vi "运维调试_其他.vi"() -> ()   [LabVIEW 2016, in "其他.lvlib"]
uses:
  <vilib>/Utility/miscctls.llb/LVPointTypeDef.ctl
  <userlib>/_SmartBalloon/Balloon Generic/Aesthetics.ctl
  <userlib>/_SmartBalloon/Balloon/Text Balloon.lvclass
  C:/Program Files (x86)/National Instruments/LabVIEW 2016/user.lib/_SmartBalloon/Balloon Generic/Balloon.lvclass
  <userlib>/_SmartBalloon/Balloon/Init Balloon.vi
  <vilib>/ptbypt/NI_PtbyPt.lvlib
  WxMessage/wxpusher.lvlib
  <userlib>/_SmartBalloon/API/SmartBalloon Library.lvclass
  <userlib>/_SmartBalloon/Balloon Generic/Balloon.lvclass
  <vilib>/Utility/config.llb/NI_LVConfig.lvlib
  update/update/update.lvlib
panel:
  in  "模块启用设置":bool
  in  "更新服务器设置":bool
  in  "站点信息设置":bool
  in  "微信通知设置":bool
  in  "定时重启":bool
  in  "首页设置":bool
  in  "短信报警设置":bool
  in  "布尔":bool
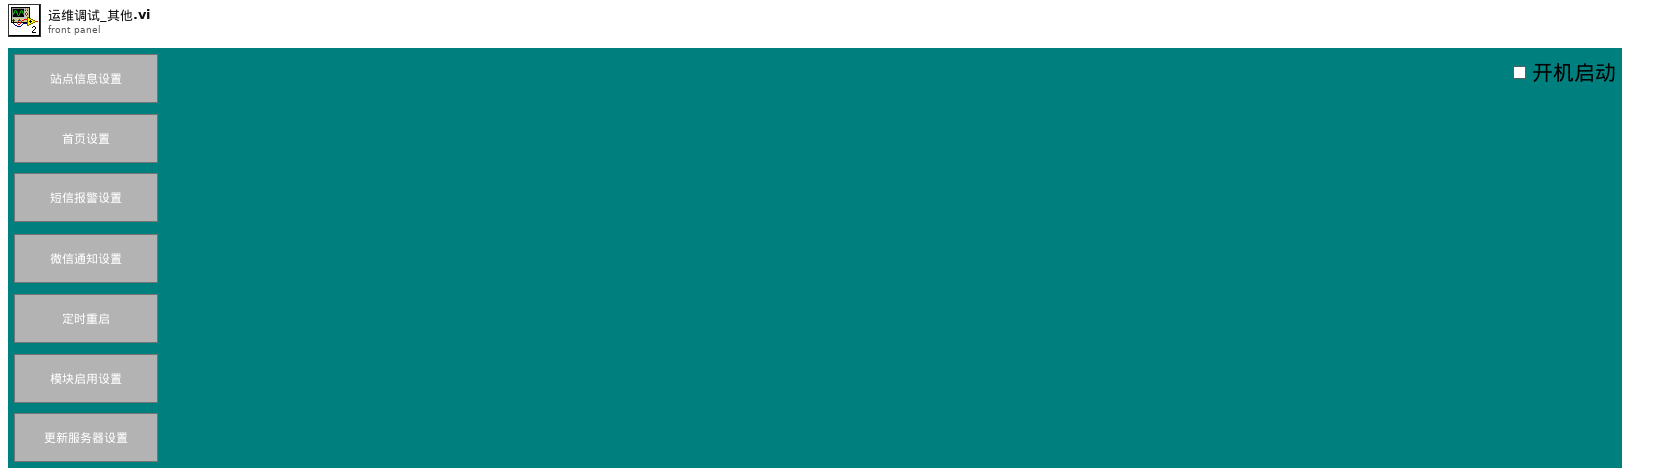
[diagram p1: front panel]
types:
  T1 = typedef "LVPointTypeDef.ctl" = cluster{"Horizontal":i16, "Vertical":i16}
  T2 = cluster{"频次":enum16{"关闭", "每天", "星期一", "星期二", "星期三", "星期四", "星期五", "星期六", "星期日"}, "时":u16, "分":u16}
  T3 = typedef "LVDateTimeRec.ctl" = cluster{"秒数的小数部分":dbl, "秒":i32, "分":i32, "时":i32, "日":i32, "月":i32, "年":i32, "天数（周）":i32, "天数（年）":i32, "DST":i32}
  T4 = enum16{"关闭", "每天", "星期一", "星期二", "星期三", "星期四", "星期五", "星期六", "星期日"}
  T5 = enum32{"Bad", "Idle", "Run top level", "Running"}
  T6 = typedef "Balloon Engine.lvlib/Balloon.lvclass/Aesthetics.ctl" = cluster{"Colors":cluster{"Font Color":u32, "Panel Color":u32}, "Display Time (ms)":i32}
  T7 = enum32{"Invalid", "Standard", "Closed", "Hidden", "Minimized", "Maximized"}
  T8 = cluster{"host":string, "user":string, "password":string, "远端地址":string}
  T9 = typedef "NI_LVConfig.lvlib/Config Data RefNum.ctl" = refnum<k1>
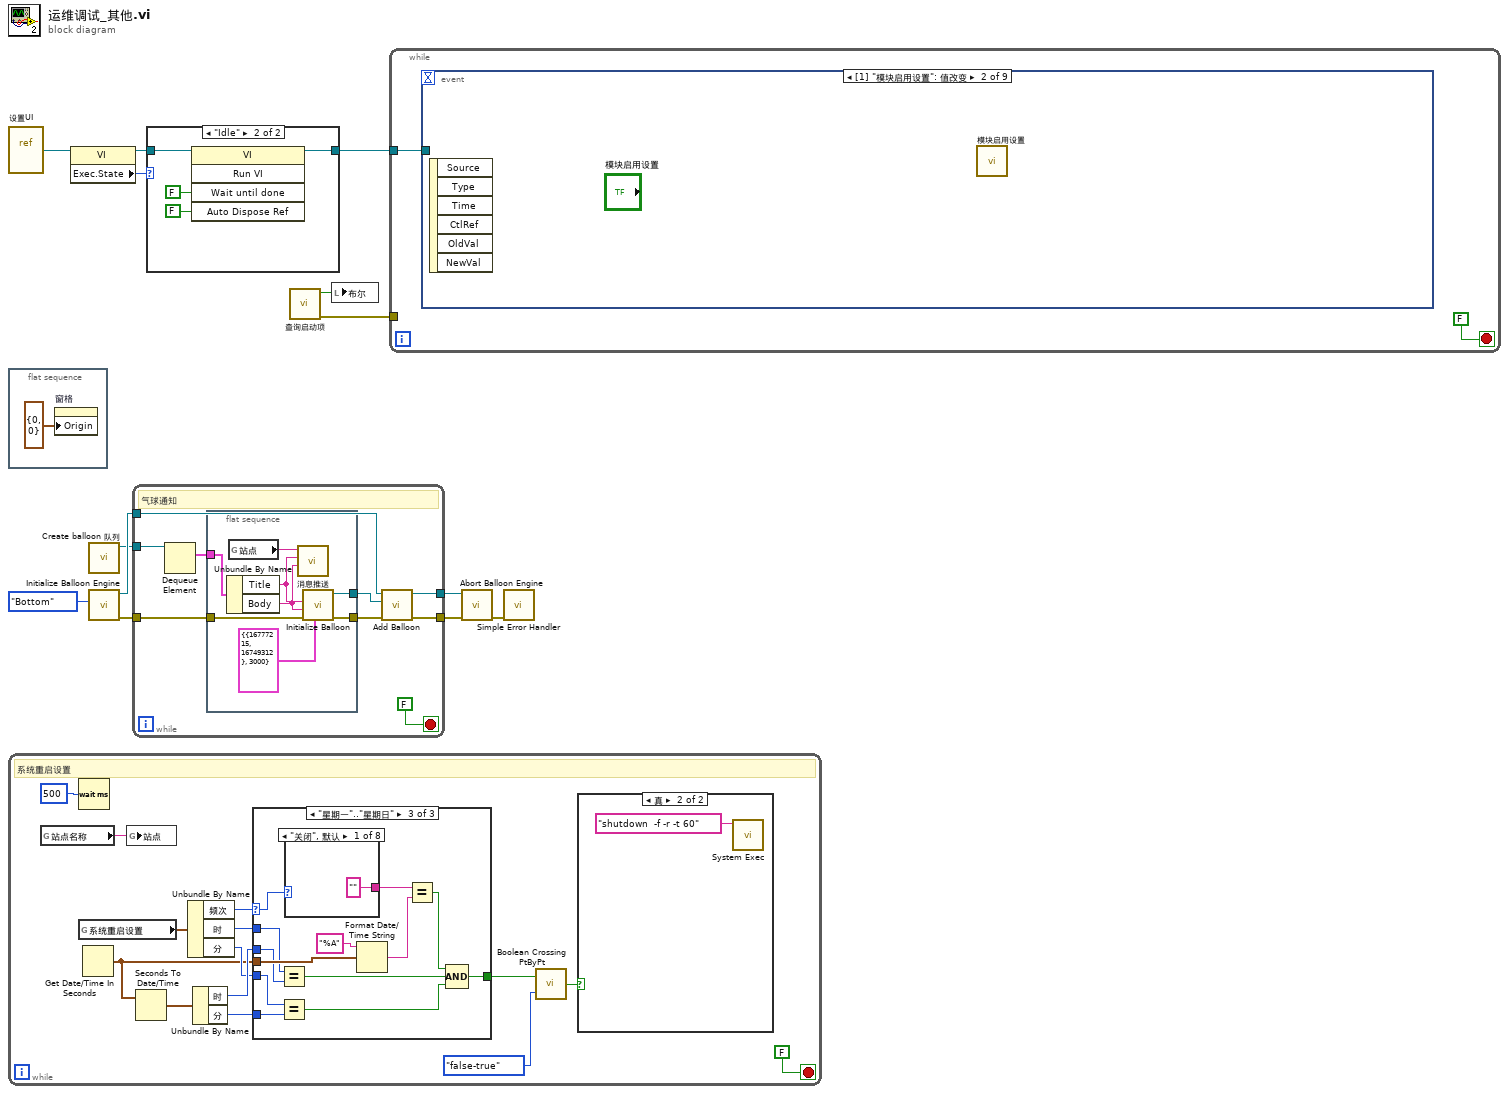
[diagram p0: block diagram]
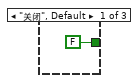
[diagram p3: hidden frame]
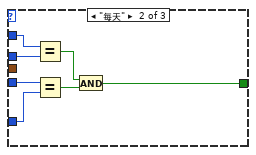
[diagram p4: hidden frame]
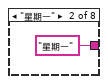
[diagram p5: hidden frame]
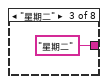
[diagram p6: hidden frame]
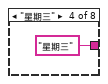
[diagram p7: hidden frame]
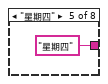
[diagram p8: hidden frame]
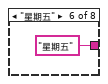
[diagram p9: hidden frame]
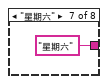
[diagram p10: hidden frame]
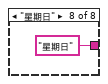
[diagram p11: hidden frame]
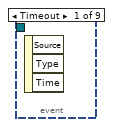
[diagram p13: hidden frame]
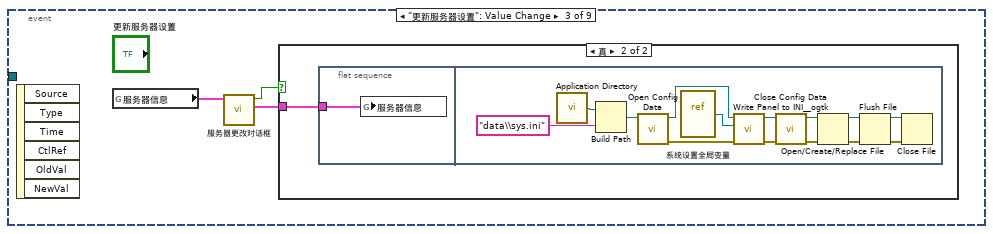
[diagram p14: hidden frame]
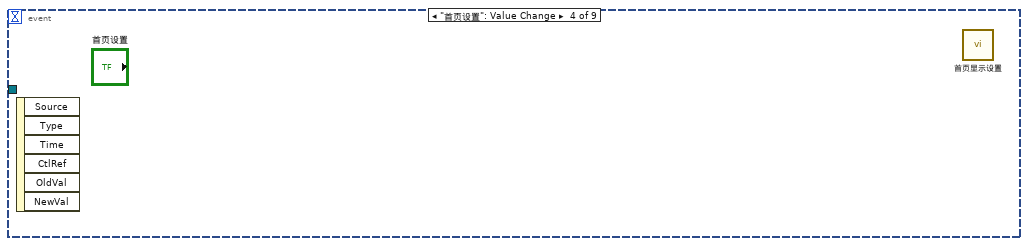
[diagram p16: hidden frame]
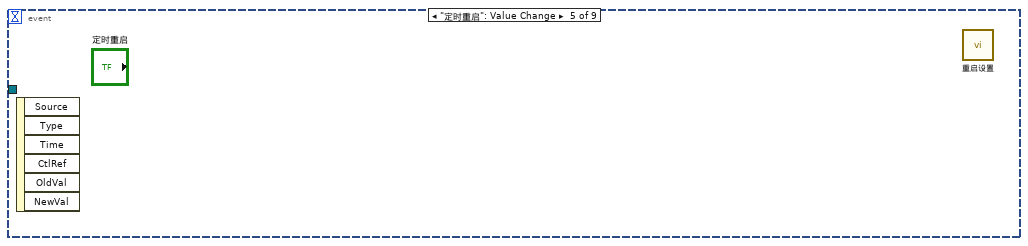
[diagram p17: hidden frame]
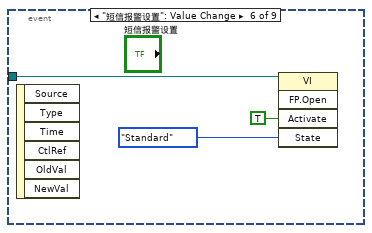
[diagram p18: hidden frame]
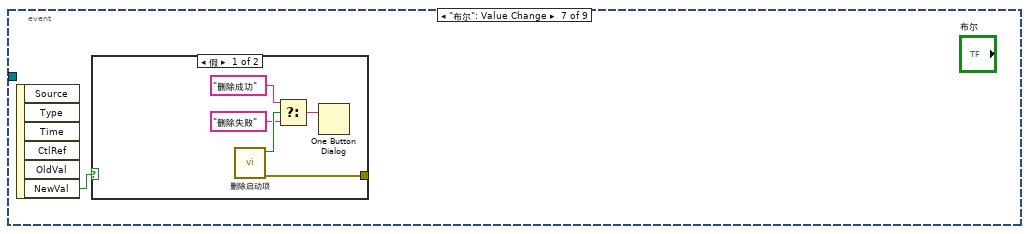
[diagram p19: hidden frame]
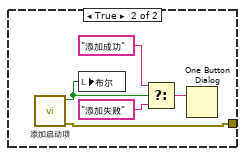
[diagram p20: hidden frame]
diagram:
  n1 = vi-ref "设置UI.vi"() -> (w11:refnum<vi>)
  n2 = flat-sequence {
    frame #0 {
      n3 = property on="窗格" class="Pane"("Origin"=T1 {"Horizontal"=0, "Vertical"=0} ("原点")) -> ()  [unwired: 2 in, 2 out]
    }
  }
  n4 = while {
    stop <- FALSE stop-if-true
    # "系统重启设置"
    n5 = global read "系统设置全局变量.vi" "站点名称"() -> (w15:string)
    n6 = Wait (ms)(milliseconds to wait=u32 500 ("等待时间（毫秒）")) -> ()  [unwired: 1 out]
    n7 = global read "系统设置全局变量.vi" "系统重启设置"() -> (w28:T2)
    n8 = Get Date/Time In Seconds() -> (seconds since 1Jan1904=w19:timestamp)
    n9 = global write "短信服务全局变量.vi" "站点"(w15) -> ()
    n10 = Seconds To Date/Time(time stamp (now)=w19) -> (date time rec=w26:T3)  [unwired: 1 in]
    n11 = Unbundle By Name(w28) -> ("频次"=w27:T4, "时"=w23:u16, "分"=w22:u16)
    n12 = Unbundle By Name(w26) -> ("时"=w25:i32, "分"=w24:i32)
    n13 = case shown="\"星期一\"..\"星期日\"" w27 {
      selector: w27 -> [_ _ w48]
      tunnel: [FALSE w31 w38] -> w18
      tunnel: w25 -> [_ w37 w42]
      tunnel: w24 -> [_ w34 w40]
      tunnel: w23 -> [_ w36 w43]
      tunnel: w22 -> [_ w35 w41]
      tunnel: w19 -> [_ _ w49]
      frame "关闭", Default {
      }
      frame "每天" {
        n14 = Equal?(x=w36, y=w37) -> (x = y?=w32:bool)
        n15 = Equal?(x=w35, y=w34) -> (x = y?=w33:bool)
        n16 = And(x=w32, y=w33) -> (x .and. y?=w31:bool)
      }
      frame "星期一".."星期日" {
        n17 = Equal?(x=w43, y=w42) -> (x = y?=w44:bool)
        n18 = Equal?(x=w41, y=w40) -> (x = y?=w45:bool)
        n19 = case shown="\"关闭\", 默认" w48 {
          tunnel: ["" ("时间格式字符串(%c)") "星期一" ("时间格式字符串(%c)") "星期二" ("时间格式字符串(%c)") "星期三" ("时间格式字符串(%c)") "星期四" ("时间格式字符串(%c)") "星期五" ("时间格式字符串(%c)") "星期六" ("时间格式字符串(%c)") "星期日" ("时间格式字符串(%c)")] -> w46
          frame "关闭", Default {
          }
          frame "星期一" {
          }
          frame "星期二" {
          }
          frame "星期三" {
          }
          frame "星期四" {
          }
          frame "星期五" {
          }
          frame "星期六" {
          }
          frame "星期日" {
          }
        }
        n20 = Format Date/Time String(time format string (%c)="%A" ("时间格式字符串(%c)"), seconds (now)=w49) -> (date/time string=w47:string)  [unwired: 1 in]
        n21 = Equal?(x=w46, y=w47) -> (x = y?=w39:bool)
        n22 = Compound Arithmetic op=AND ("复合运算")(w39, w44, w45) -> (w38:bool)
      }
    }
    n23 = call <vilib>:"Boolean Crossing PtByPt.vi"("direction"=enum16{"either", "false-true", "true-false"}."false-true", "input"=w18) -> ("crossing"=w16:bool)  [unwired: 1 in]
    n24 = case shown="真" w16 {
      frame False {
      }
      frame True {
        n25 = call <vilib>:"System Exec.vi"("command line"="shutdown  -f -r -t 60") -> ()  [unwired: 7 in, 4 out]
      }
    }
  }
  n26 = property class="VI"(reference=w11) -> (reference out=w12:refnum<vi>, "Exec.State"=w13:T5)  [unwired: 1 in, 1 out]
  n27 = call "Create balloon 队列.vi"() -> ("队列输出"=w2:refnum<queue>)  [unwired: 11 in]
  n28 = call <userlib>:"Initialize Balloon Engine.vi"("Balloon Direction"=enum16{"Top", "Bottom"}."Bottom" ("Balloon Position")) -> ("error out"=w4:errorcluster, "SmartBalloon Library.lvclass"=w7:refnum<class "SmartBalloon Library.lvclass">)  [unwired: 9 in]
  n29 = while {
    tunnel: w7 -> [w67]
    tunnel: [w66] -> w6
    tunnel: [w64] -> w5
    tunnel: w4 -> [w65]
    tunnel: w2 -> [w59]
    stop <- FALSE stop-if-true
    # "气球通知"
    n30 = Dequeue Element(queue=w59) -> (element=w60:cluster{"Title":string, "Body":string})  [unwired: 2 in, 3 out]
    n31 = flat-sequence {
      tunnel: w65 -> [w75]
      tunnel: [w74] -> w62
      tunnel: [w72] -> w61
      tunnel: w60 -> [w71]
      frame #0 {
        n32 = Unbundle By Name(w71) -> ("Title"=w70:string, "Body"=w69:string)
        n33 = global read "短信服务全局变量.vi" "站点"() -> (w68:string)
        n34 = call "消息推送.vi"("分析"=w69, "内容"=w70, "站点"=w68) -> ()  [unwired: 8 in, 1 out]
        n35 = call-poly <userlib>:"Initialize Balloon.vi"("Aesthetics"=T6 {"Colors"={"Font Color"=16777215, "Panel Color"=16749312}, "Display Time (ms)"=3000}, "error in (no error)"=w75, "Body"=w69, "Title"=w70) -> ("error out"=w72:errorcluster, "Balloon out"=w74:refnum<class "Text Balloon.lvclass">)  [unwired: 6 in]
      }
    }
    n36 = call <userlib>:"Add Balloon.vi"("error in (no error)"=w61, "Next Balloon"=w62, "SmartBalloon Engine Reference"=w67) -> ("error out"=w64:errorcluster, "SmartBalloon Engine Reference out"=w66:refnum<class "SmartBalloon Library.lvclass">)  [unwired: 7 in]
  }
  n37 = case shown="\"Idle\"" w13 {
    tunnel: w12 -> [w76 w78]
    tunnel: [w76 w77] -> w10
    frame "Bad", Default {
    }
    frame "Idle" {
      n38 = invoke class="VI" method="Run VI"(reference=w78, "Wait until done"=FALSE ("结束前等待"), "Auto Dispose Ref"=FALSE ("自动销毁引用")) -> (reference out=w77:refnum<vi>)  [unwired: 2 in, 4 out]
    }
  }
  n39 = call "查询启动项.vi"() -> ("error out"=w1:errorcluster, "包含启动项"=w9:bool)  [unwired: 10 in]
  n40 = local write "布尔"(w9) -> ()
  n41 = while {
    tunnel: w10 -> [w81]
    tunnel: w1 -> [_]
    stop <- FALSE stop-if-true
    n42 = event shown="[1] \"模块启用设置\": 值改变" {
      selector: _ -> [_ _ _ _ _ _ _ _ _]
      dyn-events: _ -> [_ _ _ _ _ _ _ _ _]
      timeout: _ -> [_ _ _ _ _ _ _ _ _]
      tunnel: w81 -> [_ _ _ _ _ w102 _ _ _]
      event Timeout {
        n43 = event-data() -> ()  [unwired: 1 in, 3 out]
      }
      event "模块启用设置": Value Change {
        n44 = event-data() -> ()  [unwired: 1 in, 6 out]
        n45 = call "模块启用设置.vi"() -> ()  [unwired: 12 in]
      }
      event "更新服务器设置": Value Change {
        n46 = event-data() -> ()  [unwired: 1 in, 6 out]
        n47 = global read "系统设置全局变量.vi" "服务器信息"() -> (w85:T8)
        n48 = call "服务器更改对话框.vi"("服务器信息"=w85) -> ("服务器信息 2"=w83:T8, "check?"=w84:bool)  [unwired: 9 in]
        n49 = case shown="真" w84 {
          tunnel: w83 -> [_ w86]
          frame False {
          }
          frame True {
            n50 = flat-sequence {
              tunnel: w86 -> [w87]
              frame #0 {
                n51 = global write "系统设置全局变量.vi" "服务器信息"(w87) -> ()
              }
              frame #1 {
                n52 = call <vilib>:"Application Directory.vi"() -> ("Application Directory"=w101:path)
                n53 = Build Path(base path=w101, name or relative path="data\\sys.ini" ("名称或相对路径")) -> (appended path=w99:path)
                n54 = call <vilib>:"Open Config Data.vi"("configuration file path"=w99) -> ("error out"=w95:errorcluster, "refnum"=w98:T9)  [unwired: 8 in, 1 out]
                n55 = vi-ref "系统设置全局变量.vi"() -> (w97:refnum<vi>)
                n56 = call <userlib>:"Write Panel to INI__ogtk.vi"("error in (no error)"=w95, "VI ref"=w97, "refnum"=w98) -> ("error out"=w94:errorcluster, "refnum out"=w96:T9)  [unwired: 7 in]
                n57 = call <vilib>:"Close Config Data.vi"("error in (no error)"=w94, "refnum"=w96) -> ("error out"=w89:errorcluster, "file path"=w88:path)  [unwired: 8 in]
                n58 = Open/Create/Replace File(file path (use dialog)=w88, error in=w89) -> (refnum out=w92:refnum<file>, error out=w93:errorcluster)  [unwired: 4 in, 1 out]
                n59 = Flush File(refnum=w92, error in=w93) -> (refnum out=w91:refnum<file>, error out=w90:errorcluster)
                n60 = Close File(refnum=w91, error in=w90) -> ()  [unwired: 2 out]
              }
            }
          }
        }
      }
      event "首页设置": Value Change {
        n61 = event-data() -> ()  [unwired: 1 in, 6 out]
        n62 = call "首页显示设置.vi"() -> ()  [unwired: 12 in]
      }
      event "定时重启": Value Change {
        n63 = event-data() -> ()  [unwired: 1 in, 6 out]
        n64 = call "重启设置.vi"() -> ()  [unwired: 12 in]
      }
      event "短信报警设置": Value Change {
        n65 = event-data() -> ()  [unwired: 1 in, 6 out]
        n66 = invoke class="VI" method="FP.Open"(reference=w102, "Activate"=TRUE ("激活？"), "State"=T7."Standard" ("状态")) -> ()  [unwired: 2 in, 5 out]
      }
      event "布尔": Value Change {
        n67 = event-data() -> ("NewVal"=w105:bool)  [unwired: 1 in, 5 out]
        n68 = case shown="假" w105 {
          tunnel: [w110 w115] -> _
          frame False {
            n69 = call "删除启动项.vi"() -> ("error out"=w110:errorcluster, "删除标记"=w109:bool)  [unwired: 10 in]
            n70 = Select(t="删除成功" ("消息"), s=w109, f="删除失败" ("消息")) -> (s? t:f=w108:string)
            n71 = One Button Dialog(message=w108) -> ()  [unwired: 1 in, 1 out]
          }
          frame True {
            n72 = call "添加启动项.vi"() -> ("error out"=w115:errorcluster, "添加成功标记"=w111:bool)  [unwired: 10 in]
            n73 = local write "布尔"(w111) -> ()
            n74 = Select(t="添加成功" ("消息"), s=w111, f="添加失败" ("消息")) -> (s? t:f=w112:string)
            n75 = One Button Dialog(message=w112) -> ()  [unwired: 1 in, 1 out]
          }
        }
      }
      event "微信通知设置": Value Change {
        n76 = event-data() -> ()  [unwired: 1 in, 6 out]
        n77 = global read "短信服务全局变量.vi" "站点"() -> (w116:string)
        n78 = call "创建参数二维码.vi"("站点"=w116) -> ()  [unwired: 11 in]
      }
      event "站点信息设置": Value Change {
        n79 = event-data() -> ()  [unwired: 1 in, 6 out]
        n80 = call "站点信息设置.vi"() -> ()  [unwired: 12 in]
      }
    }
  }
  n81 = call <userlib>:"Abort Balloon Engine.vi"("error in (no error)"=w5, "SmartBalloon Engine Reference"=w6) -> ("error out"=w3:errorcluster)  [unwired: 9 in]
  n82 = call <vilib>:"Simple Error Handler.vi"("error in (no error)"=w3) -> ()  [unwired: 4 in, 5 out]
